vi "LM Double Exponential and gradient.vi"(3 "output control":T1, 4 "data":variant, 5 "X":dbl[](array[numeric]), 6 "a":dbl[](array[numeric])) -> (0 "error out":errorcluster, 1 "f'(X,a)":dbl[][](array[numeric]), 2 "f(X,a)":dbl[](array[numeric]))   [LabVIEW 2019]
doc: "This template is the starting point for creating a model function to be passed to the Nonlinear Curve Fit.vi."
uses:
  <vilib>/gmath/NumericalOptimization/LM_output select.ctl
  <vilib>/gmath/NI_Gmath.lvlib
panel:
  # "Parameters:\n\nA1, t1\nA2, t2"
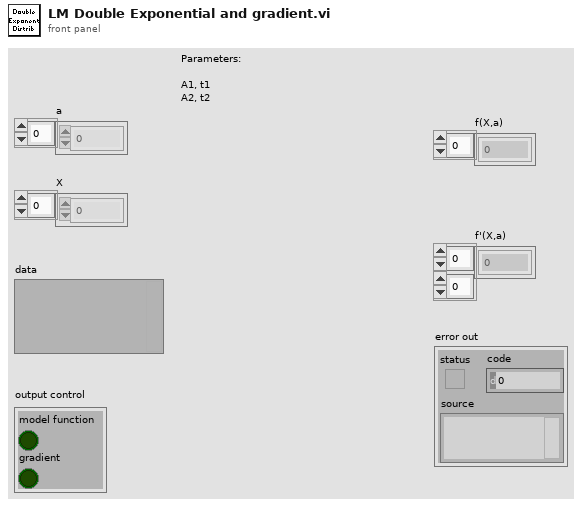
[diagram p1: front panel]
types:
  T1 = typedef "NI_Gmath.lvlib/LM_output select.ctl" = cluster{"model function":bool, "gradient":bool}
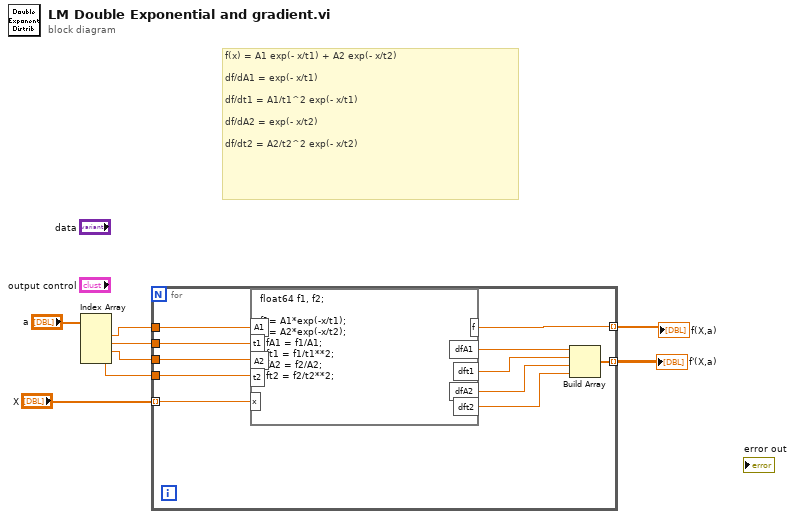
[diagram p0: block diagram]
diagram:
  # "f(x) = A1 exp(- x/t1) + A2 exp(- x/t2)\n \ndf/dA1 = exp(- x/t1)     \n\ndf/dt1 = A1/t1^2 exp(- x/t1) \n\ndf/dA2 = exp(- x/t2)     \n\ndf/dt2 = A2/t2^2 exp(- x/t2)"
  n1 = Index Array(array="a") -> (element #1=w7:dbl, element #2=w6:dbl, element #3=w5:dbl, element #4=w4:dbl)  [unwired: 4 in]
  n2 = for {
    tunnel: w7 -> [w19]
    tunnel: w6 -> [w18]
    tunnel: w5 -> [w12]
    tunnel: w4 -> [w11]
    tunnel: "X" -> [w17] mode=indexing
    tunnel: [w15] -> w2 mode=indexing
    tunnel: [w13] -> w1 mode=indexing
    n3 = formula code="float64 f1, f2;\n\nf1= A1*exp(-x/t1);\nf2= A2*exp(-x/t2);\ndfA1 = f1/A1;\ndft1 = f1/t1**2;\ndfA2 = f2/A2;\ndft2 = f2/t2**2;"("A1"=w19, "t1"=w18, "A2"=w12, "x"=w17, "t2"=w11) -> ("f"=w15:dbl, "dfA1"=w16:dbl, "dft1"=w14:dbl, "dfA2"=w10:dbl, "dft2"=w9:dbl)
    n4 = Build Array(w16, w14, w10, w9) -> (w13:dbl[])
  }
  "f(X,a)" <- w2
  "f'(X,a)" <- w1
